vi "Sub03_BilliardRect no loop.vi"(8 "error in (no error)":errorcluster, 11 "appended path":path) -> (0 "error out":errorcluster, 3 "Billard rect":T1)   [LabVIEW 2019]
panel:
  in  "Billard rect 0":T1
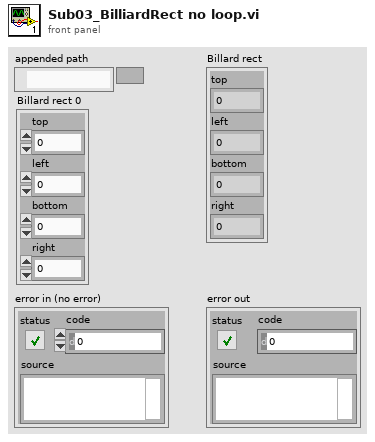
[diagram p1: front panel]
types:
  T1 = cluster{"top":dbl, "left":dbl, "bottom":dbl, "right":dbl}
  T2 = cluster{"R max":u32, "G max":u32, "B max":u32, "R min":u32, "G min":u32, "B min":u32}
  T3 = typedef "imagedata.ctl" = cluster{"image type":i32, "image depth":i32, "image":u8[], "mask":u8[], "colors":u32[], "Rectangle":cluster{"left":i16, "top":i16, "right":i16, "bottom":i16}}
  T4 = cluster{"[0]":i32, "[1]":i32, "[2]":i32, "[3]":i32, "[4]":i32, "[5]":i32, "[6]":i32, "[7]":i32, "[8]":i32}
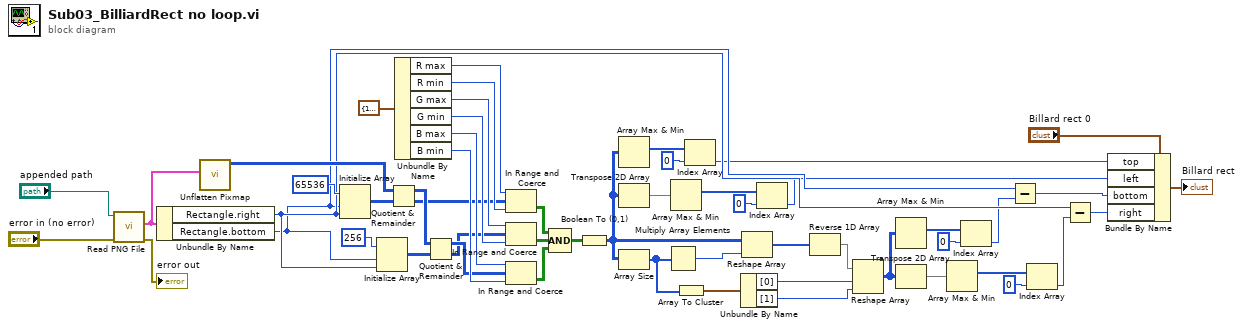
[diagram p0: block diagram]
diagram:
  n1 = call <vilib>:"Read PNG File.vi"("error in (no error)"="error in (no error)", "path to PNG file"="appended path") -> ("error out"=→"error out":errorcluster, "image data"=w53:T3)  [unwired: 7 in, 1 out]
  n2 = Unbundle By Name(w53) -> ("Rectangle.right"=w14:i16, "Rectangle.bottom"=w13:i16)
  n3 = call <vilib>:"Unflatten Pixmap.vi"("image data"=w53) -> ("24-bit pixmap"=w35:u32[][])  [unwired: 4 in, 6 out]
  n4 = Initialize Array(65536, w13, w14) -> (w36:i32[][])
  n5 = Initialize Array(256, w13, w14) -> (w37:i32[][])
  n6 = Quotient & Remainder(x=w35, y=w36) -> (x-y*floor(x/y)=w46:u32[][], floor(x/y)=w43:u32[][])
  n7 = Unbundle By Name(T2 {"R max"=14, "G max"=42, "B max"=126, "R min"=0, "G min"=0, "B min"=121} ("Colors")) -> ("R max"=w52:u32, "R min"=w51:u32, "G max"=w50:u32, "G min"=w49:u32, "B max"=w48:u32, "B min"=w47:u32)
  n8 = Quotient & Remainder(x=w46, y=w37) -> (x-y*floor(x/y)=w45:u32[][], floor(x/y)=w44:u32[][])
  n9 = In Range and Coerce(upper limit=w52, x=w43, lower limit=w51) -> (In Range?=w42:bool[][])  [unwired: 1 out]
  n10 = In Range and Coerce(upper limit=w50, x=w44, lower limit=w49) -> (In Range?=w41:bool[][])  [unwired: 1 out]
  n11 = In Range and Coerce(upper limit=w48, x=w45, lower limit=w47) -> (In Range?=w40:bool[][])  [unwired: 1 out]
  n12 = Compound Arithmetic op=AND(w42, w41, w40) -> (w34:bool[][])
  n13 = Boolean To (0,1)(Boolean=w34) -> (0, 1=w28:i16[][])
  n14 = Array Max & Min(array=w28) -> (max index (indices)=w32:i32[])  [unwired: 3 out]
  n15 = Transpose 2D Array(2D array=w28) -> (transposed array=w33:i16[][])
  n16 = Array Size(array=w28) -> (size(s)=w25:i32[])
  n17 = Multiply Array Elements(1:w25) -> (0:w24:i32)
  n18 = Array Max & Min(array=w33) -> (max index (indices)=w30:i32[])  [unwired: 3 out]
  n19 = Array To Cluster(array=w25) -> (cluster=w23:T4)
  n20 = Index Array(array=w32, index=0) -> (element=w4:i32)
  n21 = Unbundle By Name(w23) -> ("[0]"=w22:i32, "[1]"=w21:i32)
  n22 = Reshape Array(w28, w24) -> (w27:i16[])
  n23 = Index Array(array=w30, index=0) -> (element=w3:i32)
  n24 = Reverse 1D Array(array=w27) -> (reversed array=w26:i16[])
  n25 = Reshape Array(w26, w22, w21) -> (w15:i16[][])
  n26 = Array Max & Min(array=w15) -> (max index (indices)=w19:i32[])  [unwired: 3 out]
  n27 = Transpose 2D Array(2D array=w15) -> (transposed array=w20:i16[][])
  n28 = Array Max & Min(array=w20) -> (max index (indices)=w17:i32[])  [unwired: 3 out]
  n29 = Index Array(array=w19, index=0) -> (element=w11:i32)
  n30 = Subtract(x=w13, y=w11) -> (x-y=w2:i32)
  n31 = Index Array(array=w17, index=0) -> (element=w12:i32)
  n32 = Subtract(x=w14, y=w12) -> (x-y=w1:i32)
  n33 = Bundle By Name(cluster="Billard rect 0", "top"=w4, "left"=w3, "bottom"=w2, "right"=w1) -> (→"Billard rect":T1)
